vi "Array-Random element (I32).vi"(0 "Array":i32[](array[numeric])) -> (2 "Element":i32, 3 "Index":i32)   [LabVIEW 2020]
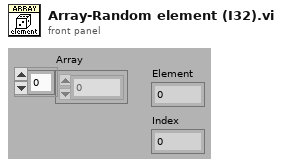
[diagram p1: front panel]
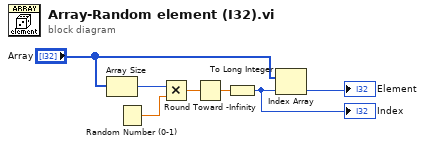
[diagram p0: block diagram]
diagram:
  n1 = Array Size(array="Array") -> (size(s)=w7:i32)
  n2 = Random Number (0-1)() -> (number: 0 to 1=w6:dbl)
  n3 = Multiply(x=w7, y=w6) -> (x*y=w5:dbl)
  n4 = Round Toward -Infinity(1:w5) -> (0:w4:dbl)
  n5 = To Long Integer(number=w4) -> (32bit integer=w3:i32)
  "Index" <- w3
  n6 = Index Array(array="Array", index=w3) -> (element=→"Element":i32)
